vi "Acquisition Message Loop.vi"(8 "error in (no error)":errorcluster, 11 "Message Queues":T1) -> (0 "error out":errorcluster)   [LabVIEW 2019, in "Acquisition.lvlib"]
doc: "Message loop for handling messages pertaining to the acquisition of data from the hardware."
uses:
  Acquisition.lvlib
  Support/Message Queue/All Message Queues.ctl
  Support/Message Queue/Message Cluster.ctl
  Controls/Data Queue.ctl
  Controls/Acquired Data.ctl
  Controls/Data Notifier.ctl
  Hardware Configuration.ctl
  Signal Type.ctl
  Acquisition State.ctl
  <vilib>/Utility/error.llb/Error Cluster From Error Code.vi
  <vilib>/ErrorRing/Error Ring.xnode
  Support/Message Queue/Message Queue.lvlib
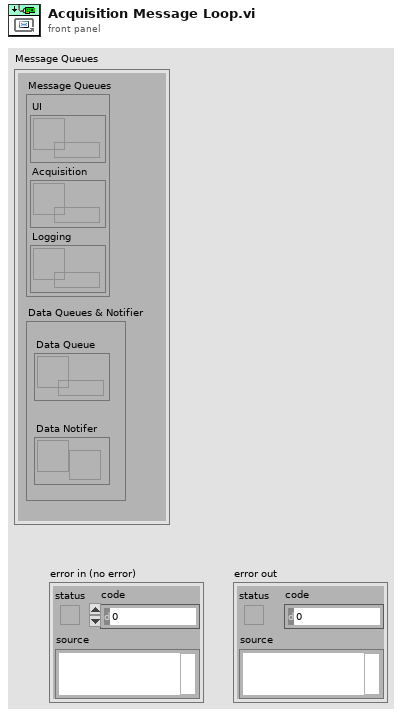
[diagram p1: front panel]
types:
  T1 = typedef "Message Queue.lvlib/All Message Queues.ctl" = cluster{"Message Queues":cluster{"UI":refnum<queue>, "Acquisition":refnum<queue>, "Logging":refnum<queue>}, "Data Queues & Notifier":cluster{"Data Queue":T2, "Data Notifer":T3}}
  T2 = typedef "Data Queue.ctl" = refnum<queue>
  T3 = typedef "Data Notifier.ctl" = refnum<notifier>
  T4 = typedef "Acquisition.lvlib/Hardware Configuration.ctl" = cluster{"HW Refnum <Replace Me>":string, "Signal Type <Replace Me>":T5}
  T5 = typedef "Acquisition.lvlib/Signal Type.ctl" = enum16{"Sine Wave", "Square with Noise"}
  T6 = typedef "Acquisition.lvlib/Acquisition State.ctl" = enum16{"Idle", "Acquiring"}
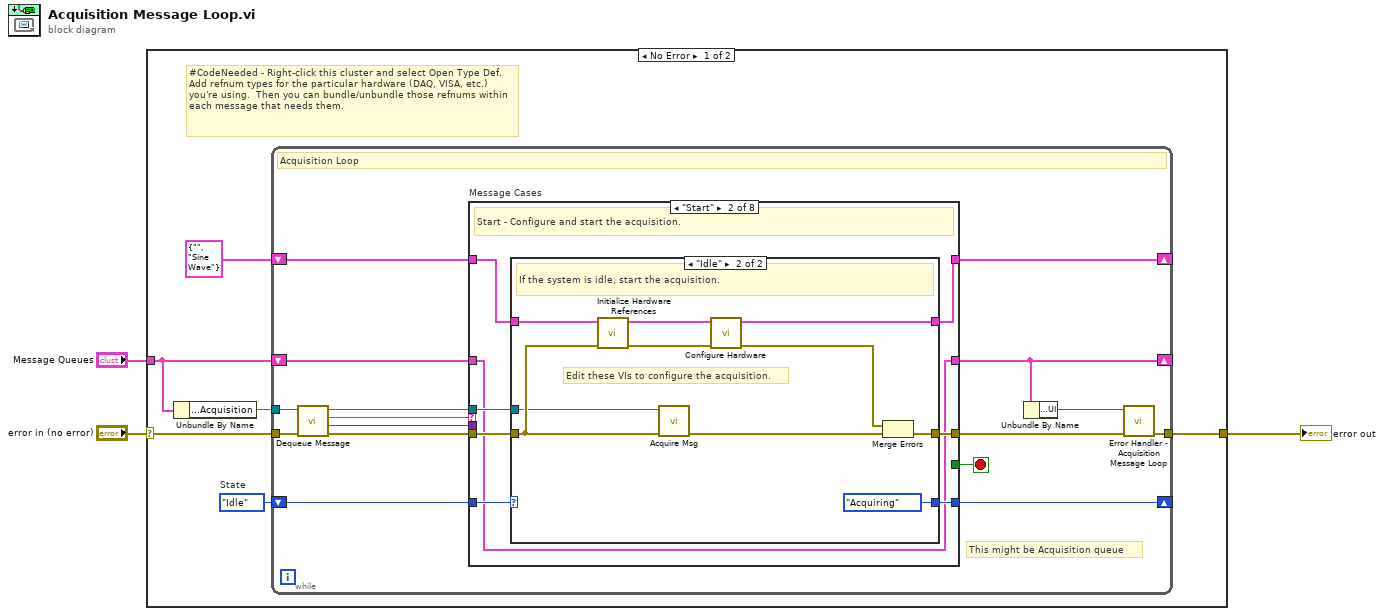
[diagram p0: block diagram]
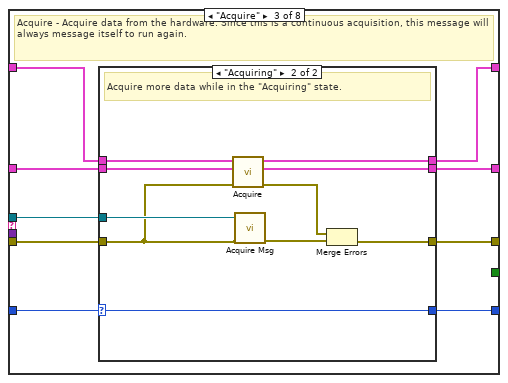
[diagram p4: hidden frame]
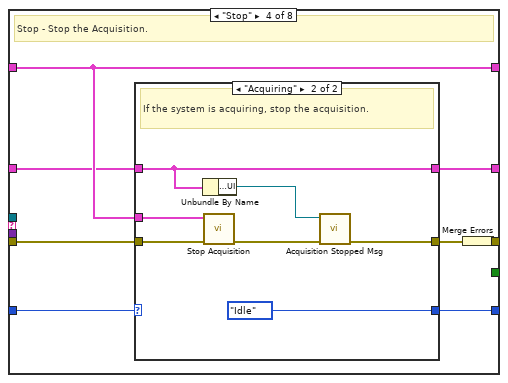
[diagram p6: hidden frame]
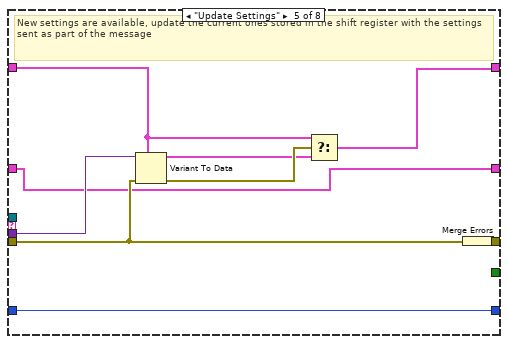
[diagram p8: hidden frame]
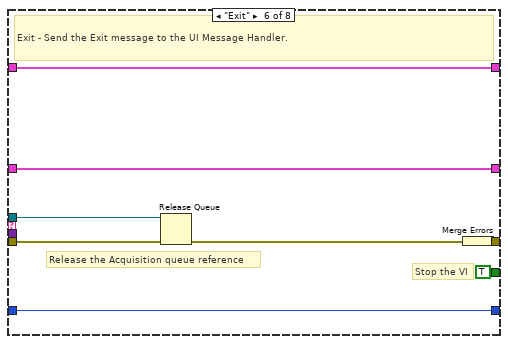
[diagram p9: hidden frame]
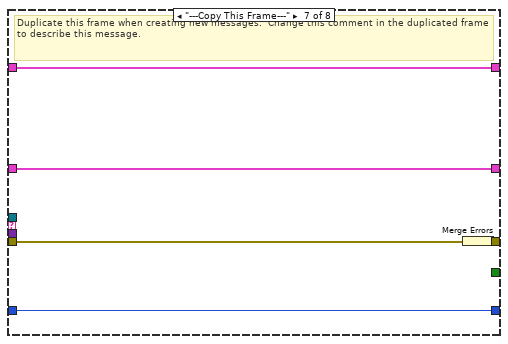
[diagram p10: hidden frame]
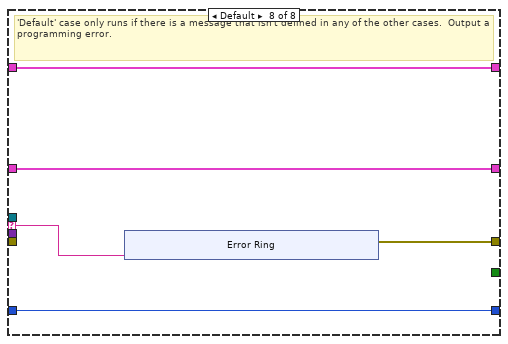
[diagram p11: hidden frame]
diagram:
  n1 = case shown="No Error" "error in (no error)" {
    selector: "error in (no error)" -> [w6 w126]
    tunnel: "Message Queues" -> [w4 _]
    tunnel: [w8 w126] -> w2
    frame No Error {
      w5 = Acquisition_State."Idle"  # State
      # "#CodeNeeded - Right-click this cluster and select Open Type Def.  Add refnum types for the particular hardware (DAQ, VISA, etc.) you're using.  Then you can bundle/unbundle those refnums within each message that needs them."
      n2 = Unbundle By Name(w4) -> ("Message Queues.Acquisition"=w9:refnum<queue>)
      n3 = while {
        tunnel: w9 -> [w18]
        shift-right: [w24] -> _
        shift-left: T4 {"HW Refnum <Replace Me>"="", "Signal Type <Replace Me>"=enum."Sine Wave"} ("Data Cluster") -> [w25]
        shift-right: [w16] -> _
        shift-left: w5 -> [w17]
        tunnel: w6 -> [w22]
        tunnel: [w15] -> w8
        shift-right: [w11] -> _
        shift-left: w4 -> [w12]
        stop <- w23 stop-if-true
        # "This might be Acquisition queue"
        # "Acquisition Loop"
        n4 = call "Dequeue Message.vi"("error in (no error)"=w22, "Message Queue"=w18) -> ("error out"=w21:errorcluster, "Message Data"=w19:variant, "Message"=w20:string, "dup Message Queue"=w13:refnum<queue>)  [unwired: 6 in]
        n5 = case "Message Cases" shown="\"Start\"" w20 {
          selector: w20 -> [_ _ _ _ _ _ _ w115]
          tunnel: w13 -> [_ w34 w58 _ _ w103 _ _]
          tunnel: w21 -> [w29 w35 w57 w80 w94 w105 w113 _]
          tunnel: [w29 w37 w59 w81 w100 w107 w111 w116] -> w14
          tunnel: w25 -> [w28 w36 w55 w78 w96 w106 w112 w118]
          tunnel: [w28 w33 w56 w78 w95 w106 w112 w118] -> w24
          tunnel: [_ _ _ _ _ TRUE _ _] -> w23
          tunnel: w19 -> [_ _ _ _ w99 _ _ _]
          tunnel: w17 -> [w27 w31 w53 w77 w93 w102 w110 w117]
          tunnel: [w27 w32 w54 w76 w93 w102 w110 w117] -> w16
          tunnel: w12 -> [w26 w30 w52 w75 w92 w101 w109 w114]
          tunnel: [w26 w30 w51 w74 w92 w101 w109 w114] -> w11
          frame "Initialize" {
            # "Initialize  - Initialize is currently a no-op.  The hardware initialization takes place in the 'Start' message."
          }
          frame "Start" {
            # "Start - Configure and start the acquisition."
            n6 = case shown="\"Idle\"" w31 {
              selector: w31 -> [w38 _]
              tunnel: [w39 w50] -> w37
              tunnel: w36 -> [w40 w49]
              tunnel: w35 -> [w39 w48]
              tunnel: w34 -> [_ w46]
              tunnel: [w40 w42] -> w33
              tunnel: [w38 Acquisition_State."Acquiring" ("Acquisition State")] -> w32
              frame "Acquiring" {
                # "The system is already acquiring. Ignore the \"Start\" message."
              }
              frame "Idle" {
                # "Edit these VIs to configure the acquisition."
                # "If the system is idle, start the acquisition."
                n7 = call "Initialize Hardware References.vi"("error in (no error)"=w48, "Hardware Resources in"=w49) -> ("error out"=w45:errorcluster, "Hardware Resources out"=w43:T4)  [unwired: 8 in]
                n8 = call "Acquire Msg.vi"("error in (no error)"=w48, "Queue in"=w46) -> ("error out"=w47:errorcluster)  [unwired: 9 in]
                n9 = call "Configure Hardware.vi"("error in (no error)"=w45, "Hardware Resources in"=w43) -> ("error out"=w44:errorcluster, "Hardware Resources out"=w42:T4)  [unwired: 8 in]
                n10 = Merge Errors(w44, w47) -> (w50:errorcluster)
              }
            }
          }
          frame "Acquire" {
            # "Acquire - Acquire data from the hardware. Since this is a continuous acquisition, this message will always message itself to run again."
            n11 = case shown="\"Acquiring\"" w53 {
              selector: w53 -> [w61 w69]
              tunnel: [w62 w73] -> w59
              tunnel: w58 -> [_ w66]
              tunnel: w57 -> [w62 w65]
              tunnel: [w63 w71] -> w56
              tunnel: w55 -> [w63 w70]
              tunnel: [w61 w69] -> w54
              tunnel: w52 -> [w60 w68]
              tunnel: [w60 w67] -> w51
              frame "Idle" {
                # "Ignore \"Acquire\" messages when the acquisition is idle."
              }
              frame "Acquiring" {
                # "Acquire more data while in the \"Acquiring\" state."
                n12 = call "Acquire.vi"("error in (no error)"=w65, "Message Queues"=w68, "Hardware Resources in"=w70) -> ("error out"=w72:errorcluster, "Message Queues out"=w67:T1, "Hardware Resources out"=w71:T4)  [unwired: 6 in]
                n13 = call "Acquire Msg.vi"("error in (no error)"=w65, "Queue in"=w66) -> ("error out"=w64:errorcluster)  [unwired: 9 in]
                n14 = Merge Errors(w72, w64) -> (w73:errorcluster)
              }
            }
          }
          frame "Stop" {
            # "Stop - Stop the Acquisition."
            n15 = case shown="\"Acquiring\"" w77 {
              selector: w77 -> [w83 _]
              tunnel: w80 -> [w84 w91]
              tunnel: [w84 w87] -> w79
              tunnel: w78 -> [_ w89]
              tunnel: [w83 Acquisition_State."Idle" ("State")] -> w76
              tunnel: w75 -> [w82 w85]
              tunnel: [w82 w85] -> w74
              frame "Idle" {
                # "The system is already idle. Ignore the \"Stop\" message."
              }
              frame "Acquiring" {
                # "If the system is acquiring, stop the acquisition."
                n16 = Unbundle By Name(w85) -> ("Message Queues.UI"=w86:refnum<queue>)
                n17 = call "Stop Acquisition.vi"("error in (no error)"=w91, "Hardware Resources in"=w89) -> ("error out"=w90:errorcluster)  [unwired: 9 in]
                n18 = call "Acquisition Stopped Msg.vi"("error in (no error)"=w90, "Queue in"=w86) -> ("error out"=w87:errorcluster)  [unwired: 9 in]
              }
            }
            n19 = Merge Errors(w79) -> (w81:errorcluster)
          }
          frame "Update Settings" {
            # "New settings are available, update the current ones stored in the shift register with the settings sent as part of the message"
            n20 = Variant To Data(error in=w94, type=w96, Variant=w99) -> (data=w97:T4, error out=w98:errorcluster)
            n21 = Select(t=w96, s=w98, f=w97) -> (s? t:f=w95:T4)
            n22 = Merge Errors(w94) -> (w100:errorcluster)
          }
          frame "Exit" {
            # "Release the Acquisition queue reference"
            # "Stop the VI"
            # "Exit - Send the Exit message to the UI Message Handler."
            n23 = Release Queue(queue=w103, error in (no error)=w105) -> (error out=w104:errorcluster)  [unwired: 1 in, 2 out]
            n24 = Merge Errors(w104) -> (w107:errorcluster)
          }
          frame "---Copy This Frame---" {
            # "Duplicate this frame when creating new messages.  Change this comment in the duplicated frame to describe this message."
            n25 = Merge Errors(w113) -> (w111:errorcluster)
          }
          frame Default {
            # "'Default' case only runs if there is a message that isn't defined in any of the other cases.  Output a programming error."
            n26 = xnode "Error Ring"("parameter 0"=w115) -> ("error out"=w116:errorcluster)
          }
        }
        n27 = Unbundle By Name(w11) -> ("Message Queues.UI"=w10:refnum<queue>)
        n28 = call "Error Handler - Acquisition Message Loop.vi"("error in (no error)"=w14, "Message Queue"=w10) -> ("dup error in"=w15:errorcluster)  [unwired: 8 in, 1 out]
      }
    }
    frame Error {
    }
  }
  "error out" <- w2
